vi "ep_Detect RVC.vi"(0 "reference voltages":dbl[](array[numeric]), 1 "RVC settings":T4, 2 "half-cycle voltage RMS":T3(array[cluster]), 3 "reset? (F)":bool, 5 "voltage flags? (F)":bool[](array[boolean]), 11 "error in (no error)":errorcluster, 12 "nominal frequency":enum16{"50 Hz", "60 Hz"}(ring), 13 "channel number":i32) -> (4 "rapid voltage changes":T2(array[cluster]), 15 "error out":errorcluster)   [LabVIEW 2014, in "NI_EP_Power Quality.lvlib"]
uses:
  <vilib>/addons/Electrical Power/PQ/NI_EP_Power Quality.lvlib
  <vilib>/addons/Electrical Power/PQ/Common/Controls/ep_Phase.ctl
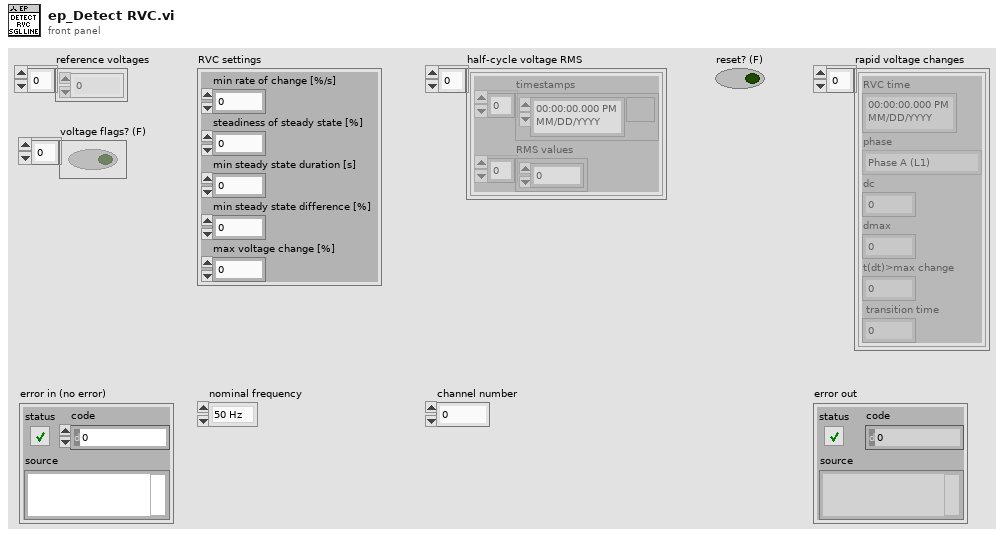
[diagram p1: front panel]
types:
  T1 = typedef "NI_EP_Power Quality.lvlib/ep_Phase.ctl" = enum16{"Phase A (L1)", "Phase B (L2)", "Phase C (L3)", "Phase N", "~3 Phases"}
  T2 = cluster{"RVC time":timestamp, "phase":T1, "dc":dbl, "dmax":dbl, "t(dt)>max change":dbl, " transition time":dbl}[]
  T3 = cluster{"timestamps":timestamp[], "RMS values":dbl[]}[]
  T4 = cluster{"min rate of change [%/s]":dbl, "steadiness of steady state [%]":dbl, "min steady state duration [s]":dbl, "min steady state difference [%]":dbl, "max voltage change [%]":dbl}
  T5 = cluster{"timestamps":timestamp[], "RMS values":dbl[]}
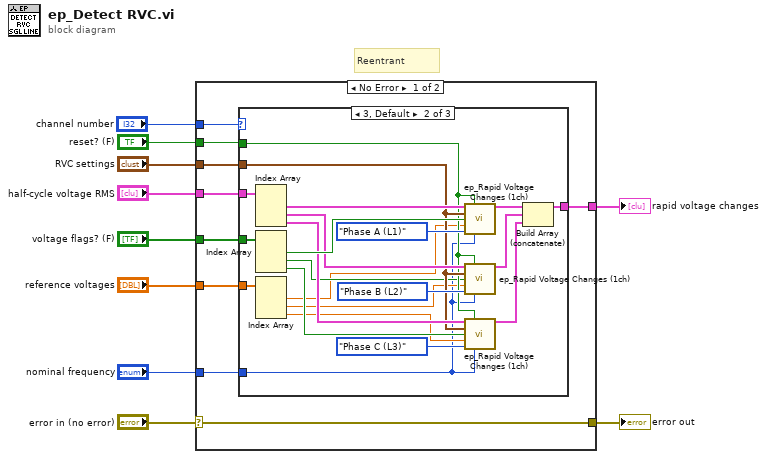
[diagram p0: block diagram]
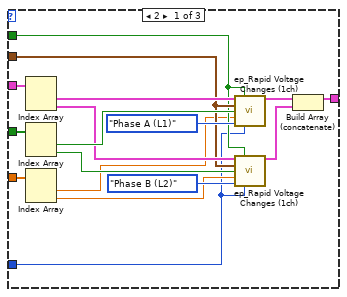
[diagram p2: hidden frame]
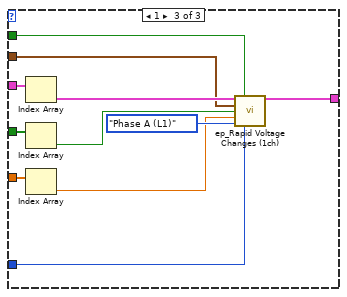
[diagram p3: hidden frame]
diagram:
  # "Reentrant"
  n1 = case shown="No Error" "error in (no error)" {
    selector: "error in (no error)" -> [w11 w70]
    tunnel: "channel number" -> [w19 _]
    tunnel: "reset? (F)" -> [w18 _]
    tunnel: "RVC settings" -> [w17 _]
    tunnel: "half-cycle voltage RMS" -> [w16 _]
    tunnel: "voltage flags? (F)" -> [w15 _]
    tunnel: "reference voltages" -> [w14 _]
    tunnel: "nominal frequency" -> [w13 _]
    tunnel: [w12 _] -> w4
    tunnel: [w11 w70] -> w2
    frame No Error {
      n2 = case shown="3, Default" w19 {
        tunnel: w16 -> [w36 w58 w69]
        tunnel: w15 -> [w35 w57 w68]
        tunnel: w17 -> [w29 w49 w63]
        tunnel: [w25 w44 w64] -> w12
        tunnel: w18 -> [w28 w48 w62]
        tunnel: w14 -> [w23 w41 w61]
        tunnel: w13 -> [w20 w37 w59]
        frame 2 {
          n3 = Index Array(array=w36) -> (element #1=w34:T5, element #2=w30:T5)  [unwired: 2 in]
          n4 = Index Array(array=w35) -> (element #1=w33:bool, element #2=w27:bool)  [unwired: 2 in]
          n5 = Index Array(array=w23) -> (element #1=w22:dbl, element #2=w21:dbl)  [unwired: 2 in]
          n6 = call <vilib>:"ep_Rapid Voltage Changes (1ch).vi"("RMS (1/2) (half cycle)"=w34, "init"=w28, "RVC settings"=w29, "voltage flag"=w33, "nominal voltage [V]"=w22, "phase"=ep_Phase."Phase A (L1)", "nominal frequency"=w20) -> ("rapid voltage changes"=w26:T2)  [unwired: 7 in, 1 out]
          n7 = call <vilib>:"ep_Rapid Voltage Changes (1ch).vi"("RMS (1/2) (half cycle)"=w30, "init"=w28, "RVC settings"=w29, "voltage flag"=w27, "nominal voltage [V]"=w21, "phase"=ep_Phase."Phase B (L2)", "nominal frequency"=w20) -> ("rapid voltage changes"=w24:T2)  [unwired: 7 in, 1 out]
          n8 = Build Array (concatenate)(w26, w24) -> (w25:T2)
        }
        frame 3, Default {
          n9 = Index Array(array=w58) -> (element #1=w56:T5, element #2=w51:T5, element #3=w50:T5)  [unwired: 3 in]
          n10 = Index Array(array=w57) -> (element #1=w55:bool, element #2=w47:bool, element #3=w46:bool)  [unwired: 3 in]
          n11 = Index Array(array=w41) -> (element #1=w40:dbl, element #2=w39:dbl, element #3=w38:dbl)  [unwired: 3 in]
          n12 = call <vilib>:"ep_Rapid Voltage Changes (1ch).vi"("RMS (1/2) (half cycle)"=w56, "init"=w48, "RVC settings"=w49, "voltage flag"=w55, "nominal voltage [V]"=w40, "phase"=ep_Phase."Phase A (L1)", "nominal frequency"=w37) -> ("rapid voltage changes"=w45:T2)  [unwired: 7 in, 1 out]
          n13 = call <vilib>:"ep_Rapid Voltage Changes (1ch).vi"("RMS (1/2) (half cycle)"=w51, "init"=w48, "RVC settings"=w49, "voltage flag"=w47, "nominal voltage [V]"=w39, "phase"=ep_Phase."Phase B (L2)", "nominal frequency"=w37) -> ("rapid voltage changes"=w43:T2)  [unwired: 7 in, 1 out]
          n14 = call <vilib>:"ep_Rapid Voltage Changes (1ch).vi"("RMS (1/2) (half cycle)"=w50, "init"=w48, "RVC settings"=w49, "voltage flag"=w46, "nominal voltage [V]"=w38, "phase"=ep_Phase."Phase C (L3)", "nominal frequency"=w37) -> ("rapid voltage changes"=w42:T2)  [unwired: 7 in, 1 out]
          n15 = Build Array (concatenate)(w45, w43, w42) -> (w44:T2)
        }
        frame 1 {
          n16 = Index Array(array=w69) -> (element=w67:T5)  [unwired: 1 in]
          n17 = Index Array(array=w68) -> (element=w66:bool)  [unwired: 1 in]
          n18 = Index Array(array=w61) -> (element=w60:dbl)  [unwired: 1 in]
          n19 = call <vilib>:"ep_Rapid Voltage Changes (1ch).vi"("RMS (1/2) (half cycle)"=w67, "init"=w62, "RVC settings"=w63, "voltage flag"=w66, "nominal voltage [V]"=w60, "phase"=ep_Phase."Phase A (L1)", "nominal frequency"=w59) -> ("rapid voltage changes"=w64:T2)  [unwired: 7 in, 1 out]
        }
      }
    }
    frame Error {
    }
  }
  "rapid voltage changes" <- w4
  "error out" <- w2
